vi "Fix Broken Rule.vi"(10 "Rule":i32[](array[numeric]), 11 "Page":i32[](array[numeric])) -> (2 "Fixed Out":bool, 3 "Page Out":i32[](array[numeric]))   [LabVIEW 2024]
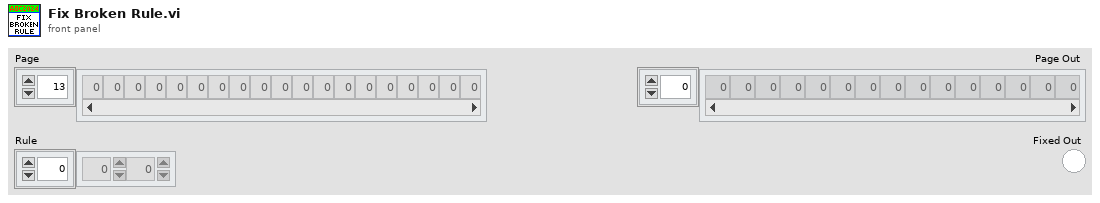
[diagram p1: front panel]
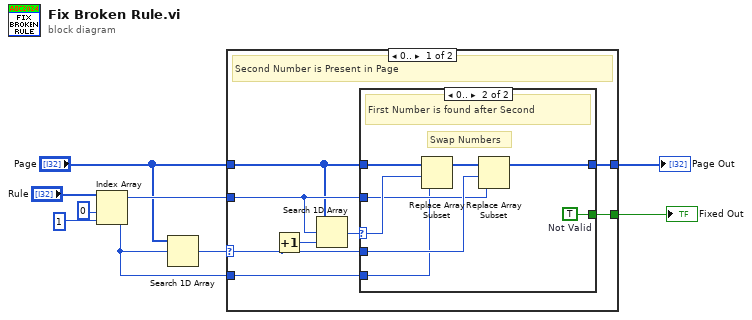
[diagram p0: block diagram]
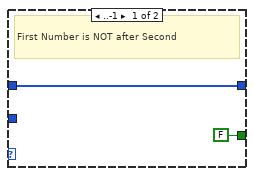
[diagram p2: hidden frame]
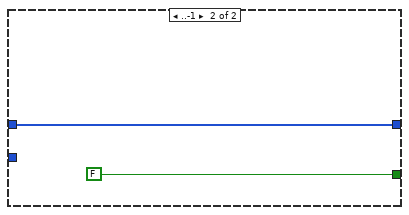
[diagram p3: hidden frame]
diagram:
  n1 = Index Array(array="Rule", index #1=0 ("index"), index #2=1 ("index")) -> (element #1=w6:i32, element #2=w9:i32)
  n2 = Search 1D Array(1D array="Page", element=w9) -> (index of element=w4:i32)  [unwired: 1 in]
  n3 = case shown="0.." w4 {
    selector: w4 -> [w12 _]
    tunnel: "Page" -> [w10 w28]
    tunnel: w6 -> [w13 _]
    tunnel: [w16 FALSE ("Not Valid")] -> w7
    tunnel: [w15 w28] -> w8
    tunnel: w9 -> [w14 _]
    frame 0.. {
      # "Second Number is Present in Page"
      n4 = Increment(x=w12) -> (x+1=w11:i32)
      n5 = Search 1D Array(1D array=w10, element=w13, start index (0)=w11) -> (index of element=w17:i32)
      n6 = case shown="0.." w17 {
        selector: w17 -> [_ w23]
        tunnel: w12 -> [_ w22]
        tunnel: [FALSE ("Not Valid") w27] -> w16
        tunnel: w13 -> [_ w21]
        tunnel: w10 -> [w18 w26]
        tunnel: [w18 w24] -> w15
        tunnel: w14 -> [_ w20]
        frame ..-1 {
          # "First Number is NOT after Second"
        }
        frame 0.. {
          w27 = TRUE  # Not Valid
          # "Swap Numbers"
          # "First Number is found after Second"
          n7 = Replace Array Subset(array=w26, new element=w20, index=w23) -> (w25:i32[])
          n8 = Replace Array Subset(array=w25, new element=w21, index=w22) -> (w24:i32[])
        }
      }
    }
    frame ..-1 {
    }
  }
  "Page Out" <- w8
  "Fixed Out" <- w7
